vi "Get DDGIOC Frequency.vi"(11 "frequency":dbl) -> (2 "function return":u32, 3 "frequency out":dbl)   [LabVIEW 2018, in "Copy of Andor SDK.lvlib"]
doc: "EXPNETTYPE unsigned int WINAPI GetDDGIOCFrequency(double * frequency);"
uses:
  Copy of Andor SDK.lvlib
  <userlib>/Andor SDK/ATMCD32D.dll
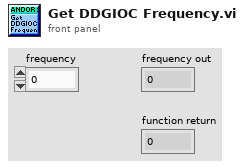
[diagram p1: front panel]
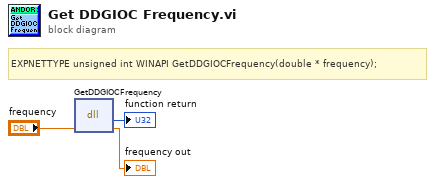
[diagram p0: block diagram]
diagram:
  # "EXPNETTYPE unsigned int WINAPI GetDDGIOCFrequency(double * frequency);"
  n1 = dll-call lib="C:/Program Files (x86)/National Instruments/LabVIEW 2018/user.lib/Andor SDK/ATMCD32D.*" fn="GetDDGIOCFrequency"("frequency"="frequency") -> (→"function return":u32, "frequency"=→"frequency out":dbl)  [unwired: 3 in, 2 out]
